vi "go2 -o.vi"() -> ()   [LabVIEW 2016]
uses:
  Classes/Controller/Motion/A3200 Folder/A3200.lvclass
  D:/Gantry_General/Classes/Controller/Motion/Motion Folder/Motion.lvclass
  Classes/Controller/Dispenser/Ultimus V2 Folder/Ultimus V2.lvclass
  Classes/Controller/I-O/NI-DAQ Folder/NI-DAQ.lvclass
  Classes/Controller/Motion/Motion Folder/Motion.lvclass
  Classes/Controller/I-O/I-O Folder/I-O.lvclass
  Classes/Controller/Dispenser/Dispenser Folder/Dispenser.lvclass
  <vilib>/Utility/file.llb/Read Delimited Spreadsheet (DBL).vi
panel:
  in  "controller in":T1
  out "draw point Cluster":T2
  in  "go patten":bool
  in  "tool go":bool
  in  "Tab Control":T3(tab)
  in  "XY go":bool
  in  "Z move to zero":bool
  in  "gule distances":dbl[](array[numeric])=[-0.6]
  out "needle XYZTheta In":dbl[](array[numeric])=[735.0, 1000.0, 55.0, 0.0]
  in  "needle xy":dbl[](array[numeric])=[735.0, 1000.0]
  in  "move to needle position":bool
  in  "XY":dbl[](array[numeric])=[1209.23, 800.59]
  in  "Camera to assembly center":bool
  in  "Camera sensor center":dbl[](array[numeric])=[1017.9301336735598, 802.7343660518175]
  in  "Camera to sensor center":bool
  in  "sensor angle":dbl=0.574830155359412
  in  "get sensor center":bool
  in  "get assembly center":bool
  in  "Syringe offset":dbl[](array[numeric])=[-219.555, -67.964]
  in  "Camera assembly center":dbl[](array[numeric])=[988.4421979205747, 1092.915302669506]
  in  "Syringe to assembly center":bool
  out "Syringe CAD center":dbl[](array[numeric])=[768.8871979205746, 1024.951302669506]
  in  "assembly angle":dbl=0.8050892331369087
  in  "get Syringe offset":bool
  in  "P0 on Delay":dbl=0.3 caption="Delay Time (s)"
  in  "new/data":bool
  in  "Vacuum Setting (0000)":i64 min=0 max=1000 step=1 format="%04.0f"
  in  "dispense change status":bool
  in  "Pressure":i16=30
  in  "on Delay":dbl=0.3 caption="Delay Time (s)"
  in  "off time":dbl=500.0
  in  "y":dbl=1.0
  out "delay off time":dbl=0.839
  in  "IO on /off":bool
  in  "Indices":i32[](array[numeric])=[11]
  in  "Values":bool[](array[boolean])=[FALSE]
  out "subarray":bool[](array[boolean])
  in  "baseplate thickness":dbl
  in  "Gule thickness":dbl
  in  "Sensor thickness":dbl
  in  "tool height":dbl
  in  "PCB thickness":dbl
  in  "file path (dialog if empty)":path=path "D:/Gantry_General/Main/ms_kao/data/CAD patten/CAD PCB full 0.8 P30 20210608/CAD PCB full 0.8 P30 20210608.txt"
  in  "Z height":dbl
  out "save data path":path=path "D:/Gantry_General/Main/ms_kao/data/CAD patten/CAD PCB full 0.8 P30 20210608/time/time20210712-164503.825.txt"
  out "folder and file name Cluster":T4={"Path"=path "D:/Gantry_General/Main/ms_kao/data/CAD patten/CAD PCB full 0.8 P30 20210608", "folder name"="time", "file name"="time", "extension"="txt", "add time string"=FALSE}
  out "i":i32=74
  out "size(s)":i32=75
  in  "stop":bool
  in  "go CAD":bool
  in  "new/data speed":bool
  in  "XY new Speed":dbl=25.0
  # "點膠速度"
  # "設定新速度"
  # "使用新/資料速度"
  # "間距70 mm"
  # "(1050, 865)\n(1050, 935)\n(1050,1005)"
  # "(910, 865)\n(910, 935)\n(910,1005)"
  # "(980, 865)\n(980, 935)\n(980,1005)"
  # "(840, 865)\n(840, 935)\n(840,1005)"
  # "9.5mm"
  # "0.32mm"
  # "0.2mm"
  # "0.1mm"
  # "0.1mm"
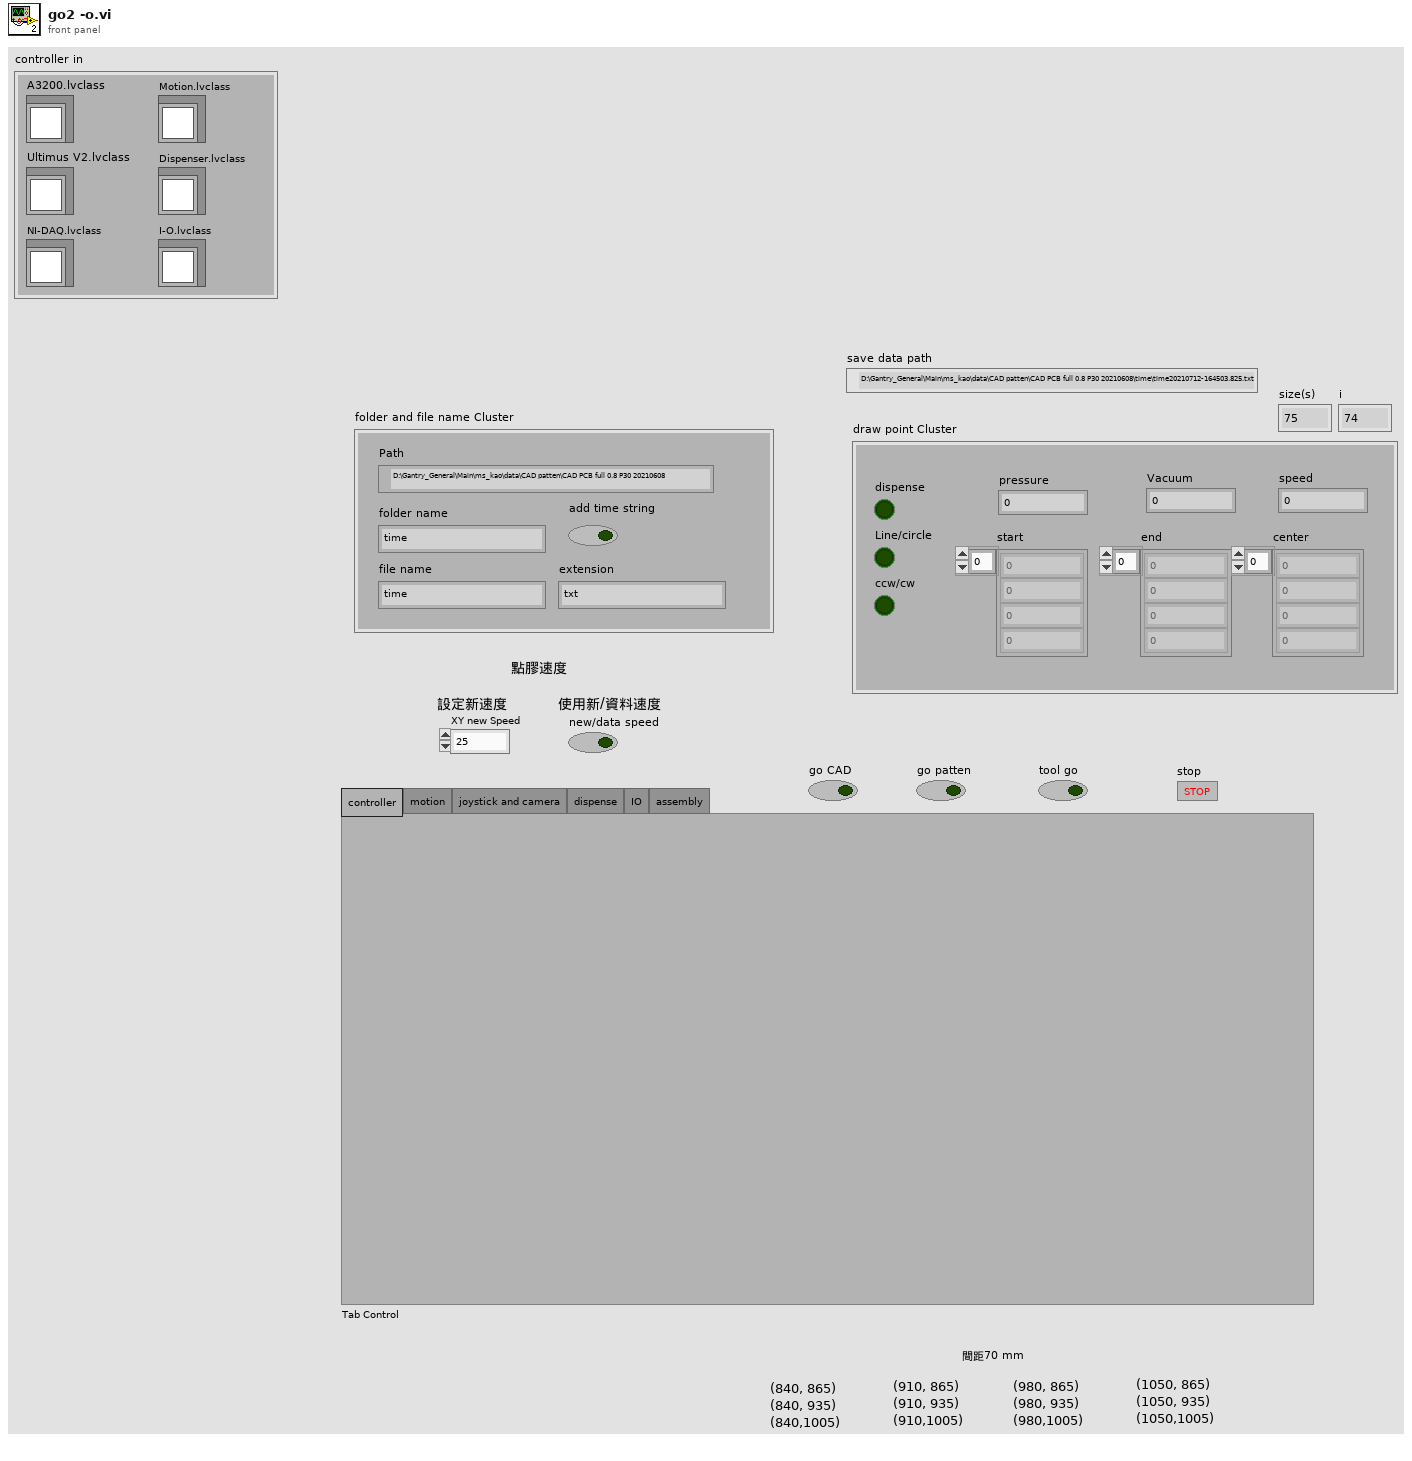
[diagram p1: front panel]
types:
  T1 = cluster{"A3200.lvclass":refnum<class "A3200.lvclass">, "Ultimus V2.lvclass":refnum<class "Ultimus V2.lvclass">, "NI-DAQ.lvclass":refnum<class "NI-DAQ.lvclass">, "Motion.lvclass":refnum<class "Motion.lvclass">, "I-O.lvclass":refnum<class "I-O.lvclass">, "Dispenser.lvclass":refnum<class "Dispenser.lvclass">}
  T2 = cluster{"dispense":bool, "Line/circle":bool, "ccw/cw":bool, "pressure":dbl, "speed":dbl, "start":dbl[], "end":dbl[], "center":dbl[], "Vacuum":dbl}
  T3 = enum32{"controller", "motion", "joystick and camera", "dispense", "IO", "assembly"}
  T4 = cluster{"Path":path, "folder name":string, "file name":string, "extension":string, "add time string":bool}
  T5 = cluster{"dispense":bool, "Line/circle":bool, "ccw/cw":bool, "pressure":dbl, "speed":dbl, "start":dbl[], "end":dbl[], "center":dbl[], "Vacuum":dbl}[]
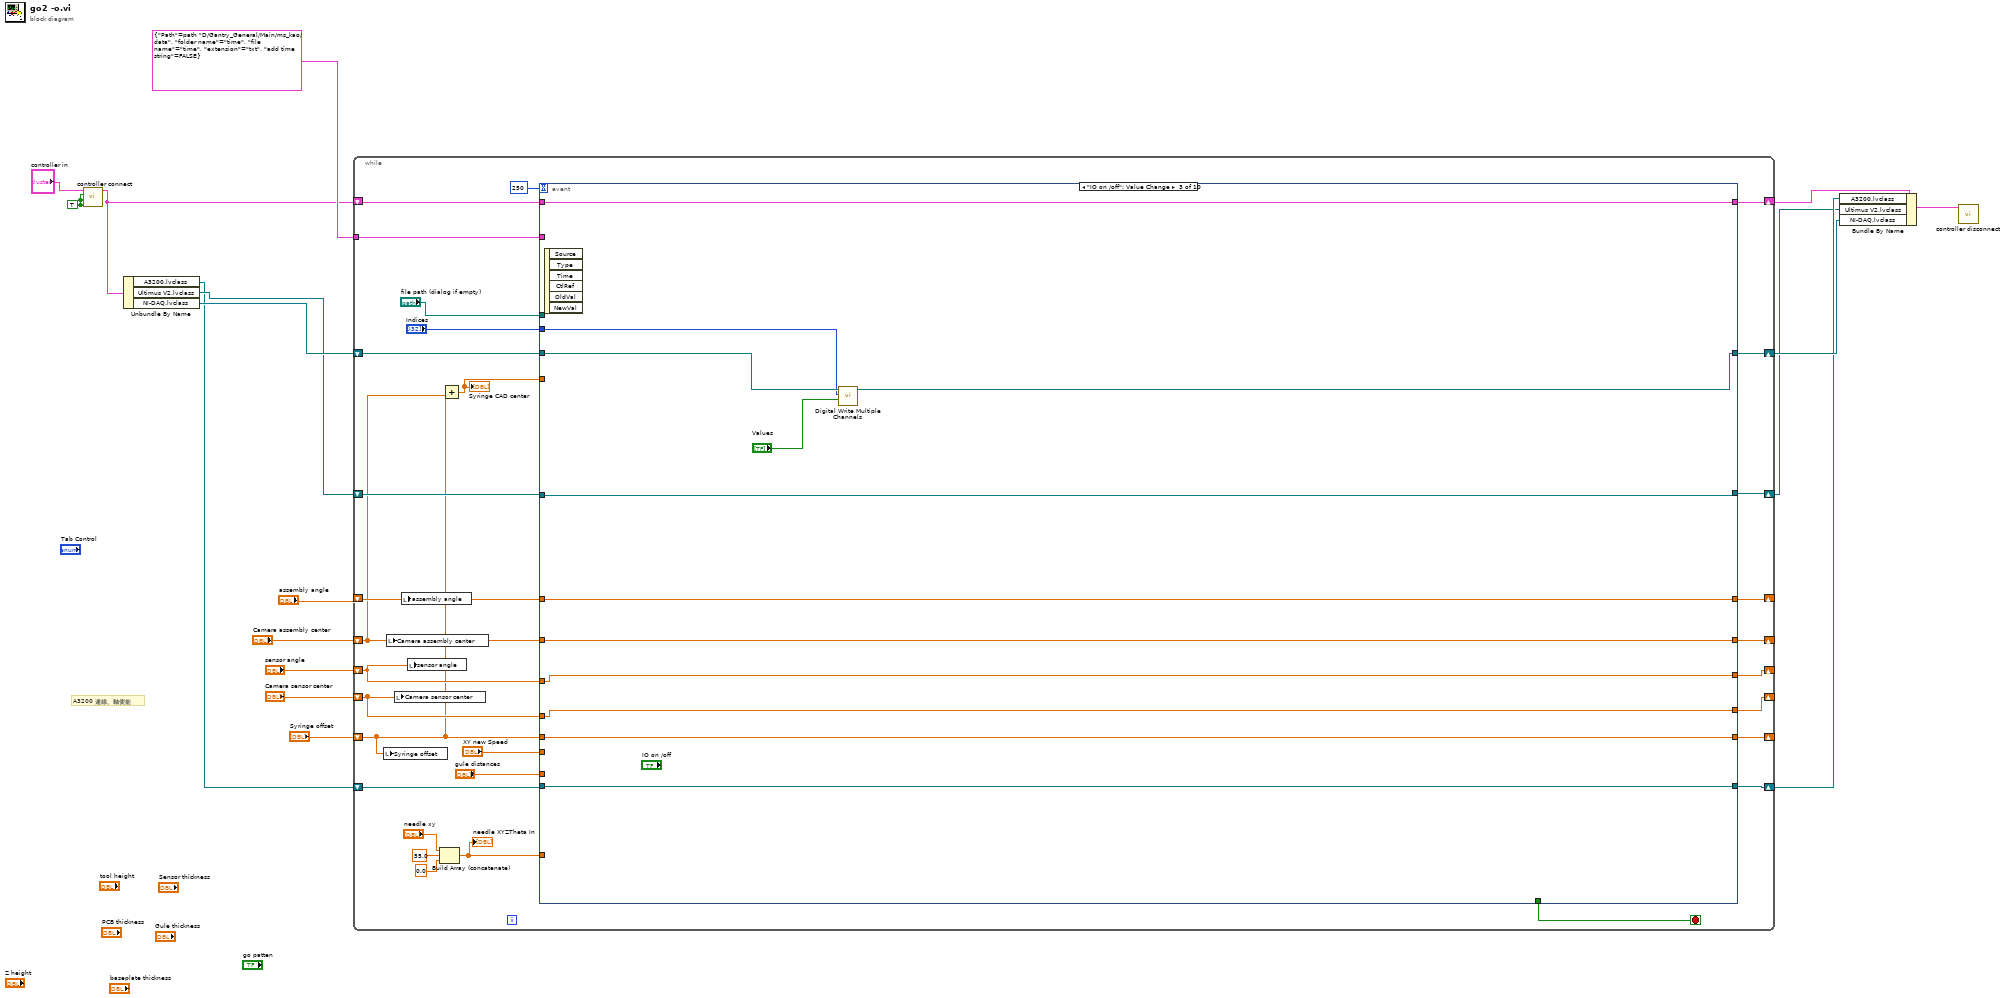
[diagram p0: block diagram]
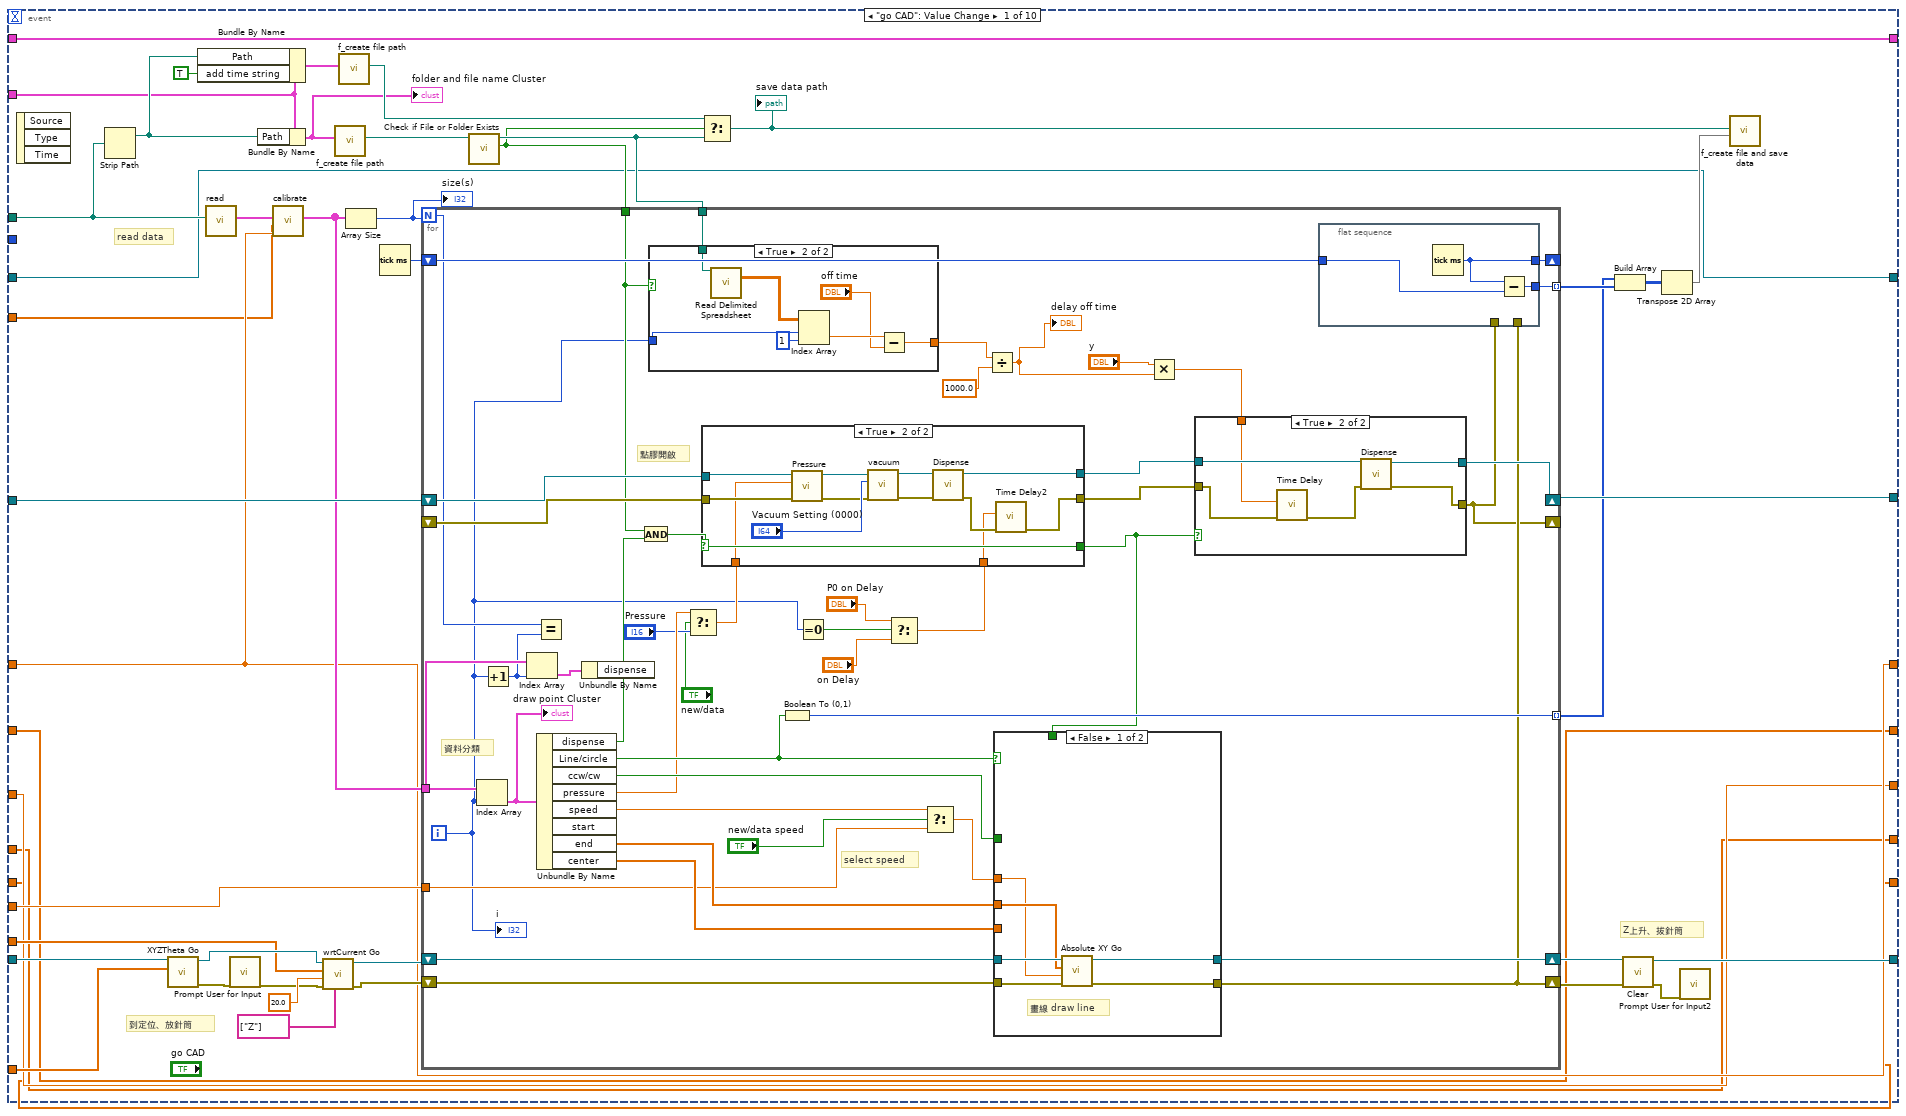
[diagram p2: hidden frame]
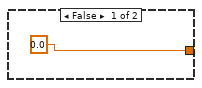
[diagram p3: hidden frame]
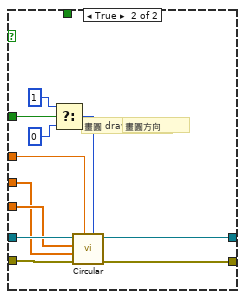
[diagram p6: hidden frame]
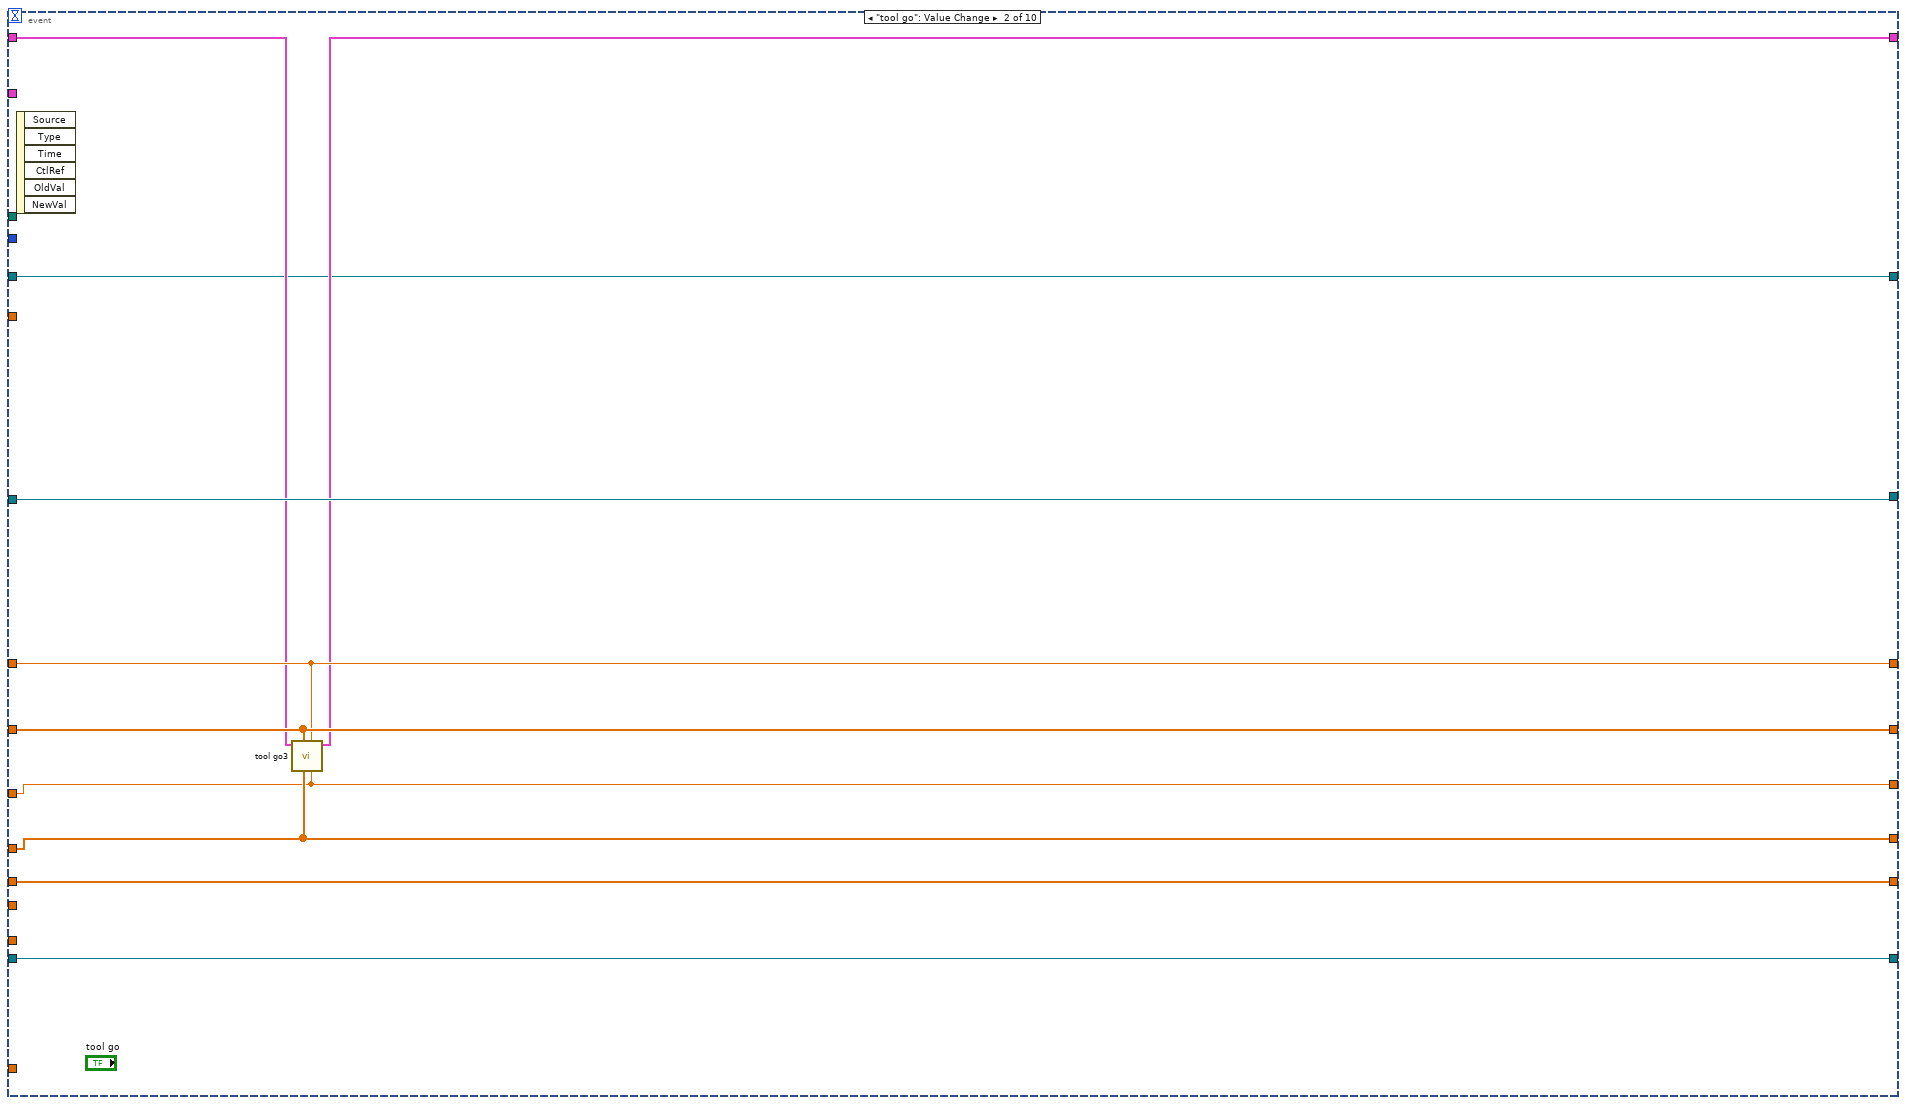
[diagram p7: hidden frame]
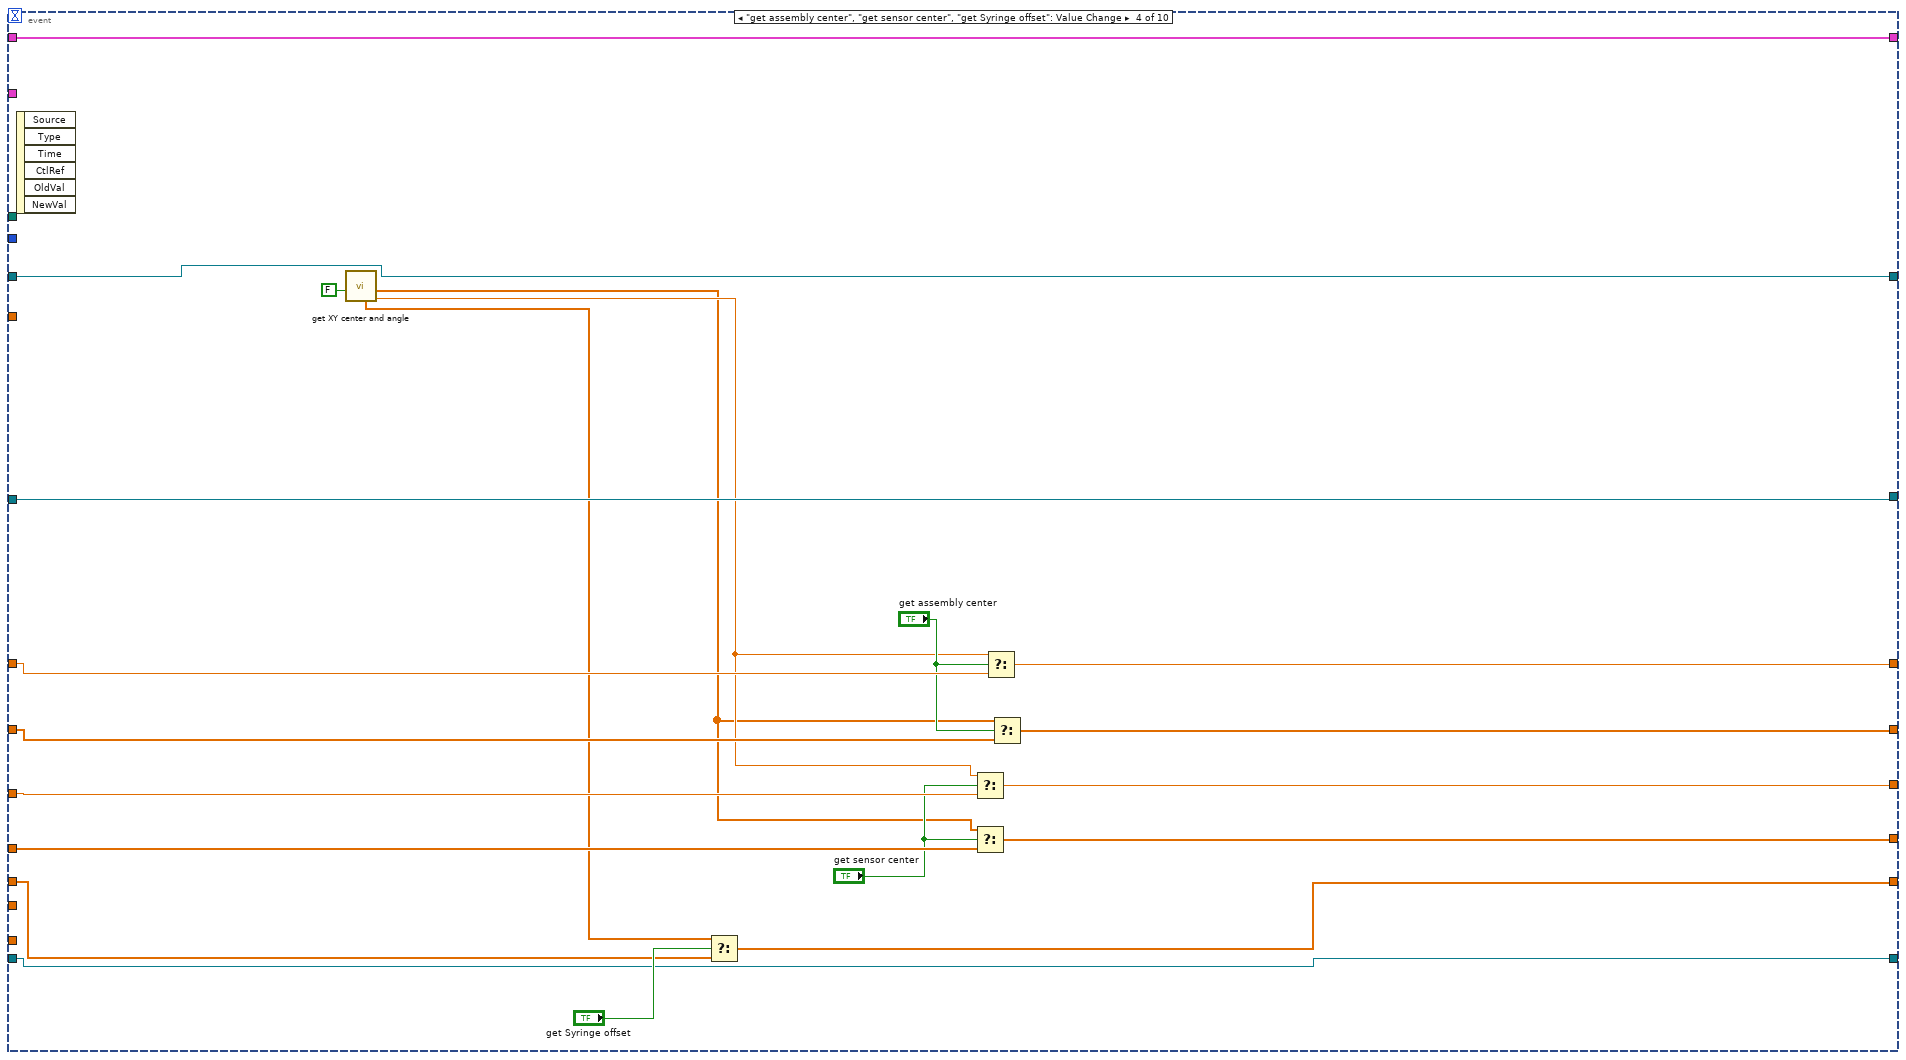
[diagram p8: hidden frame]
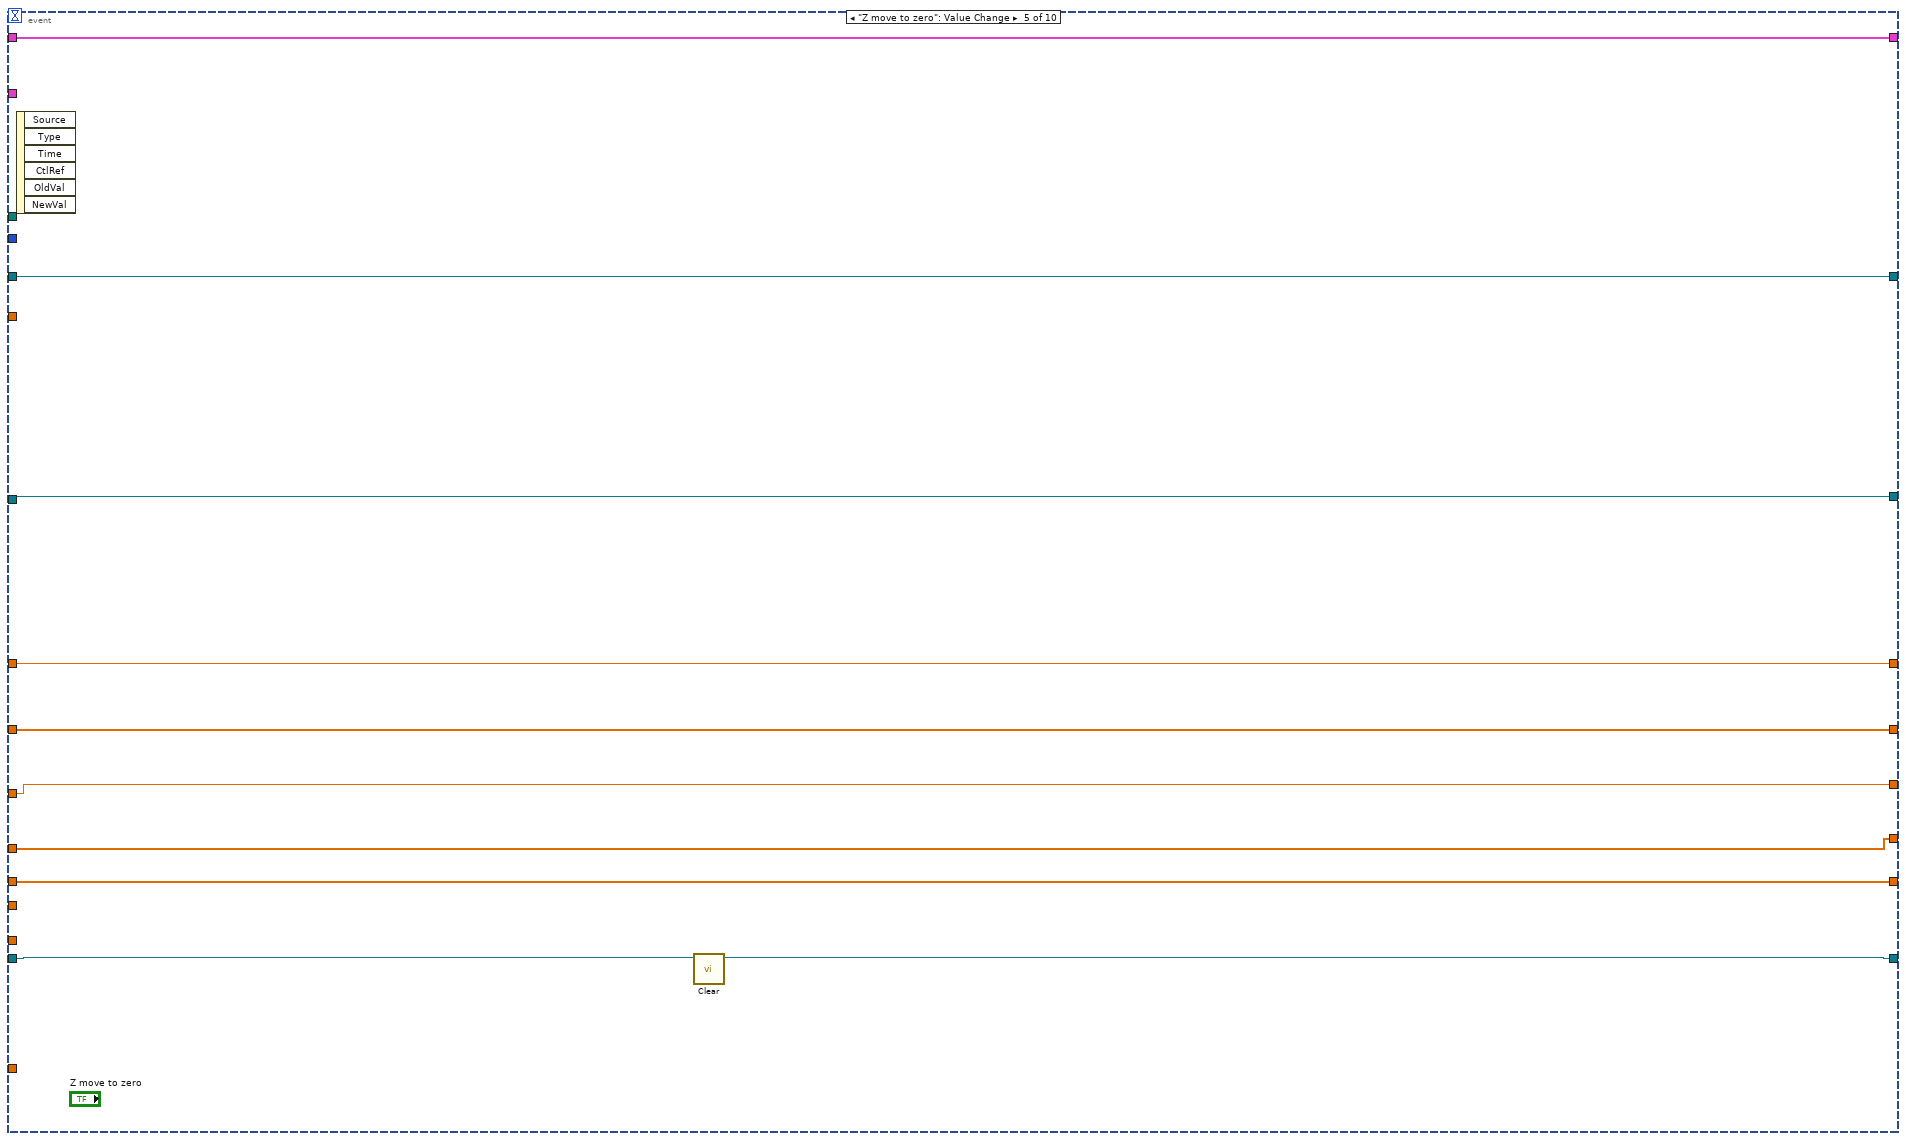
[diagram p9: hidden frame]
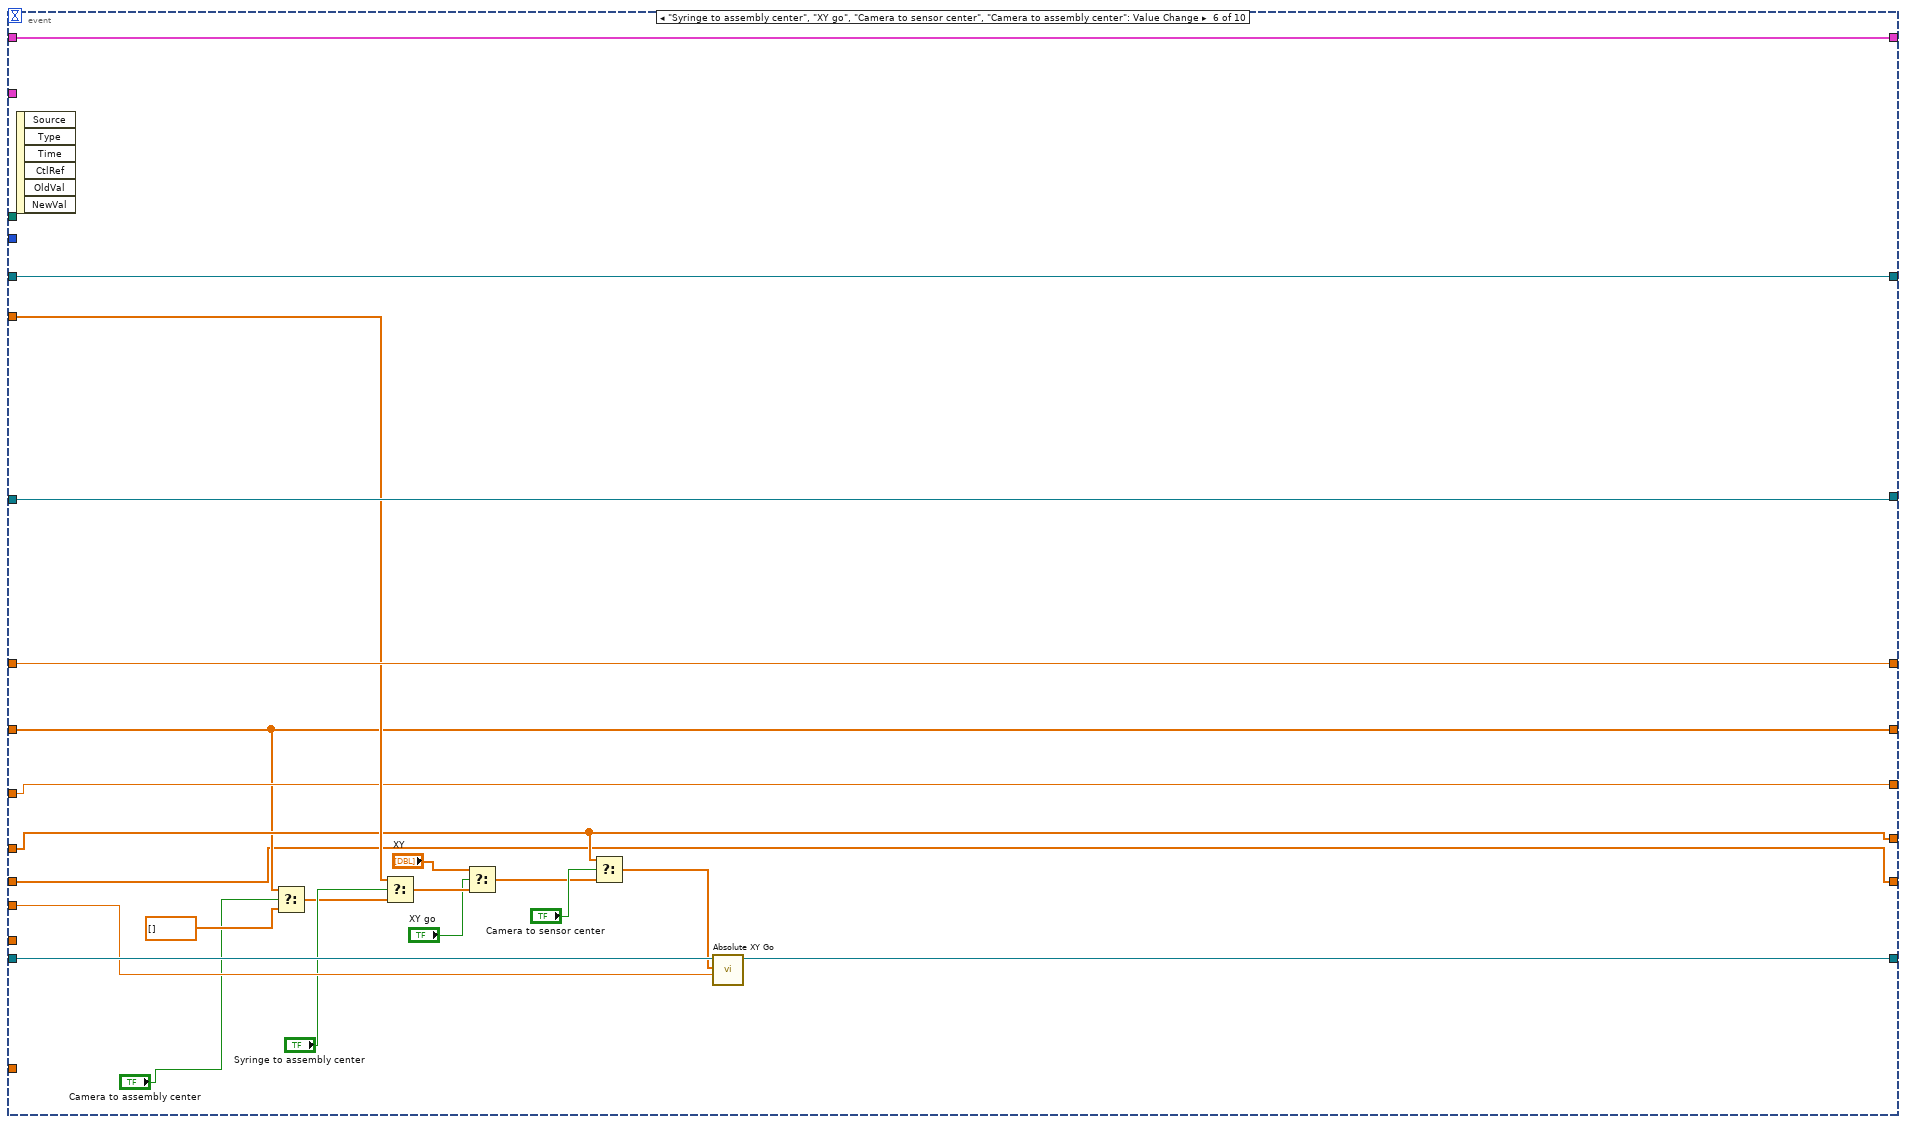
[diagram p10: hidden frame]
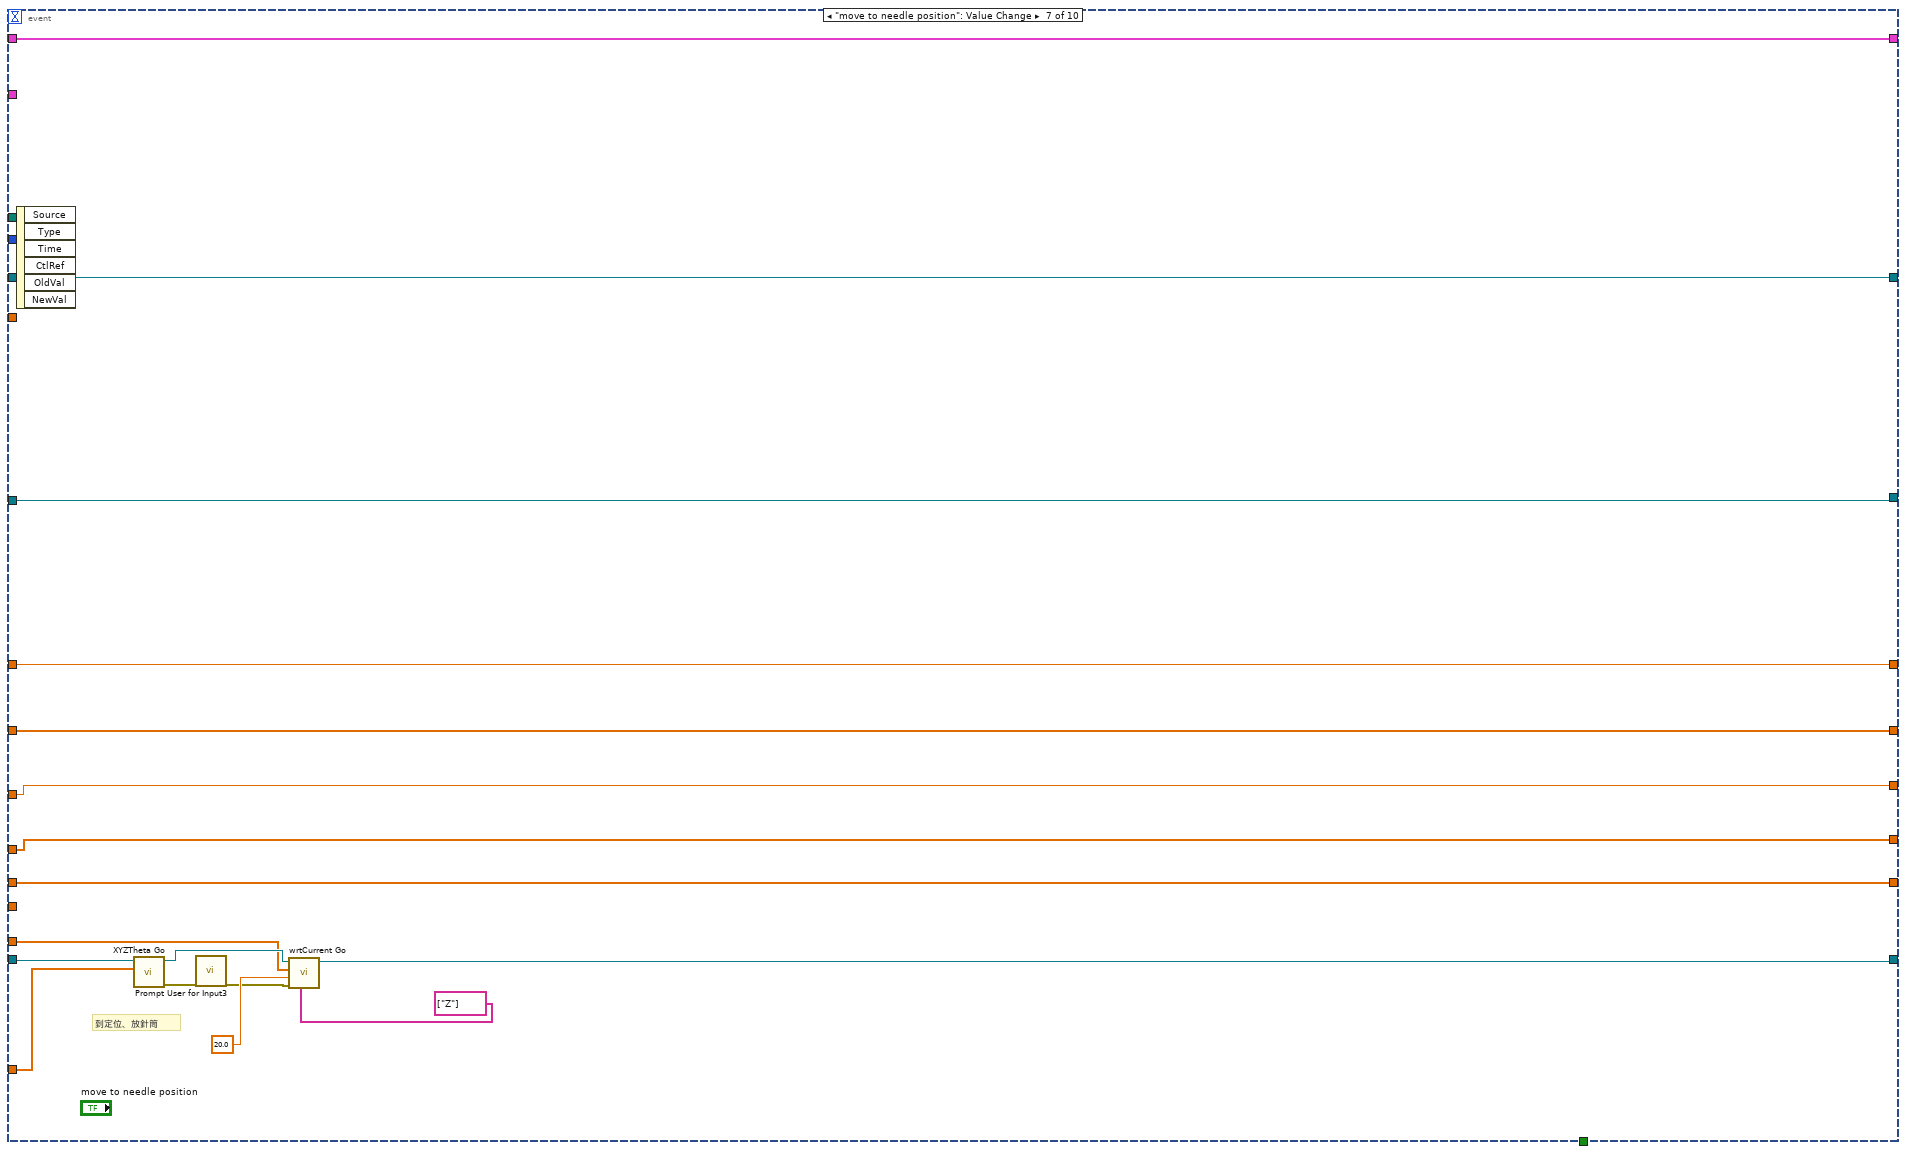
[diagram p11: hidden frame]
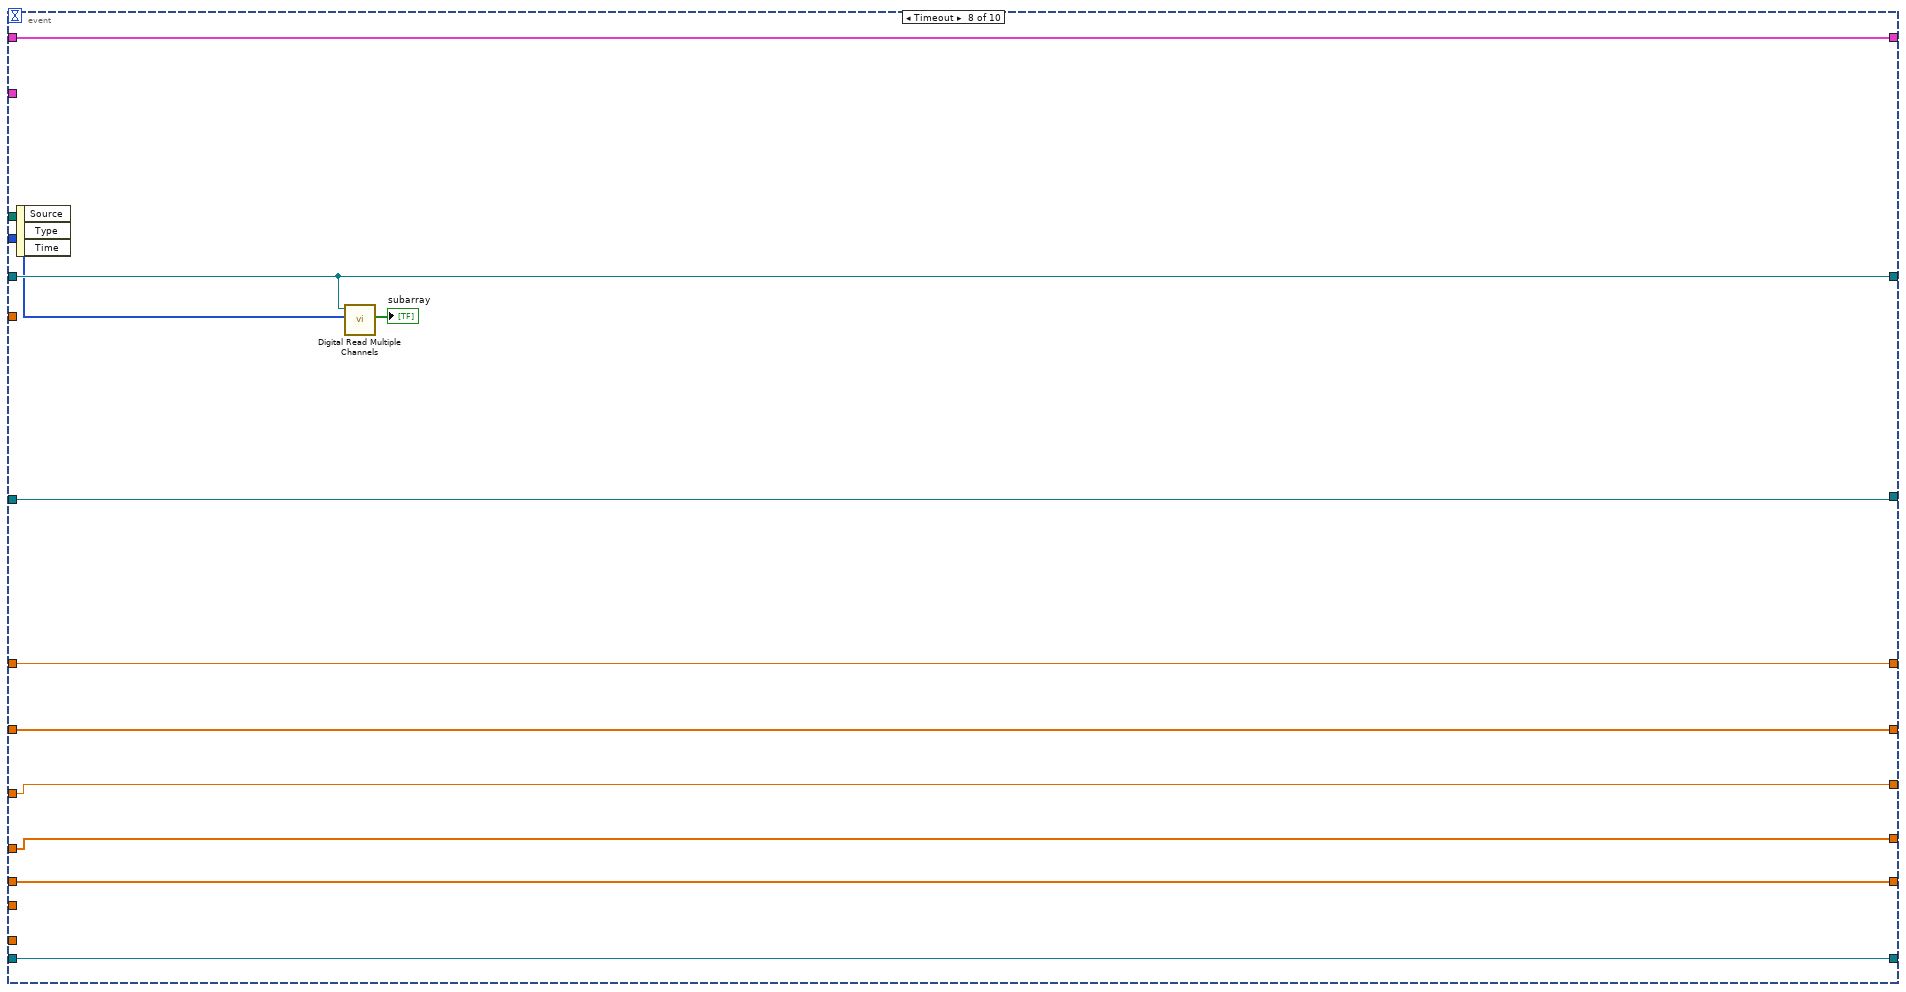
[diagram p12: hidden frame]
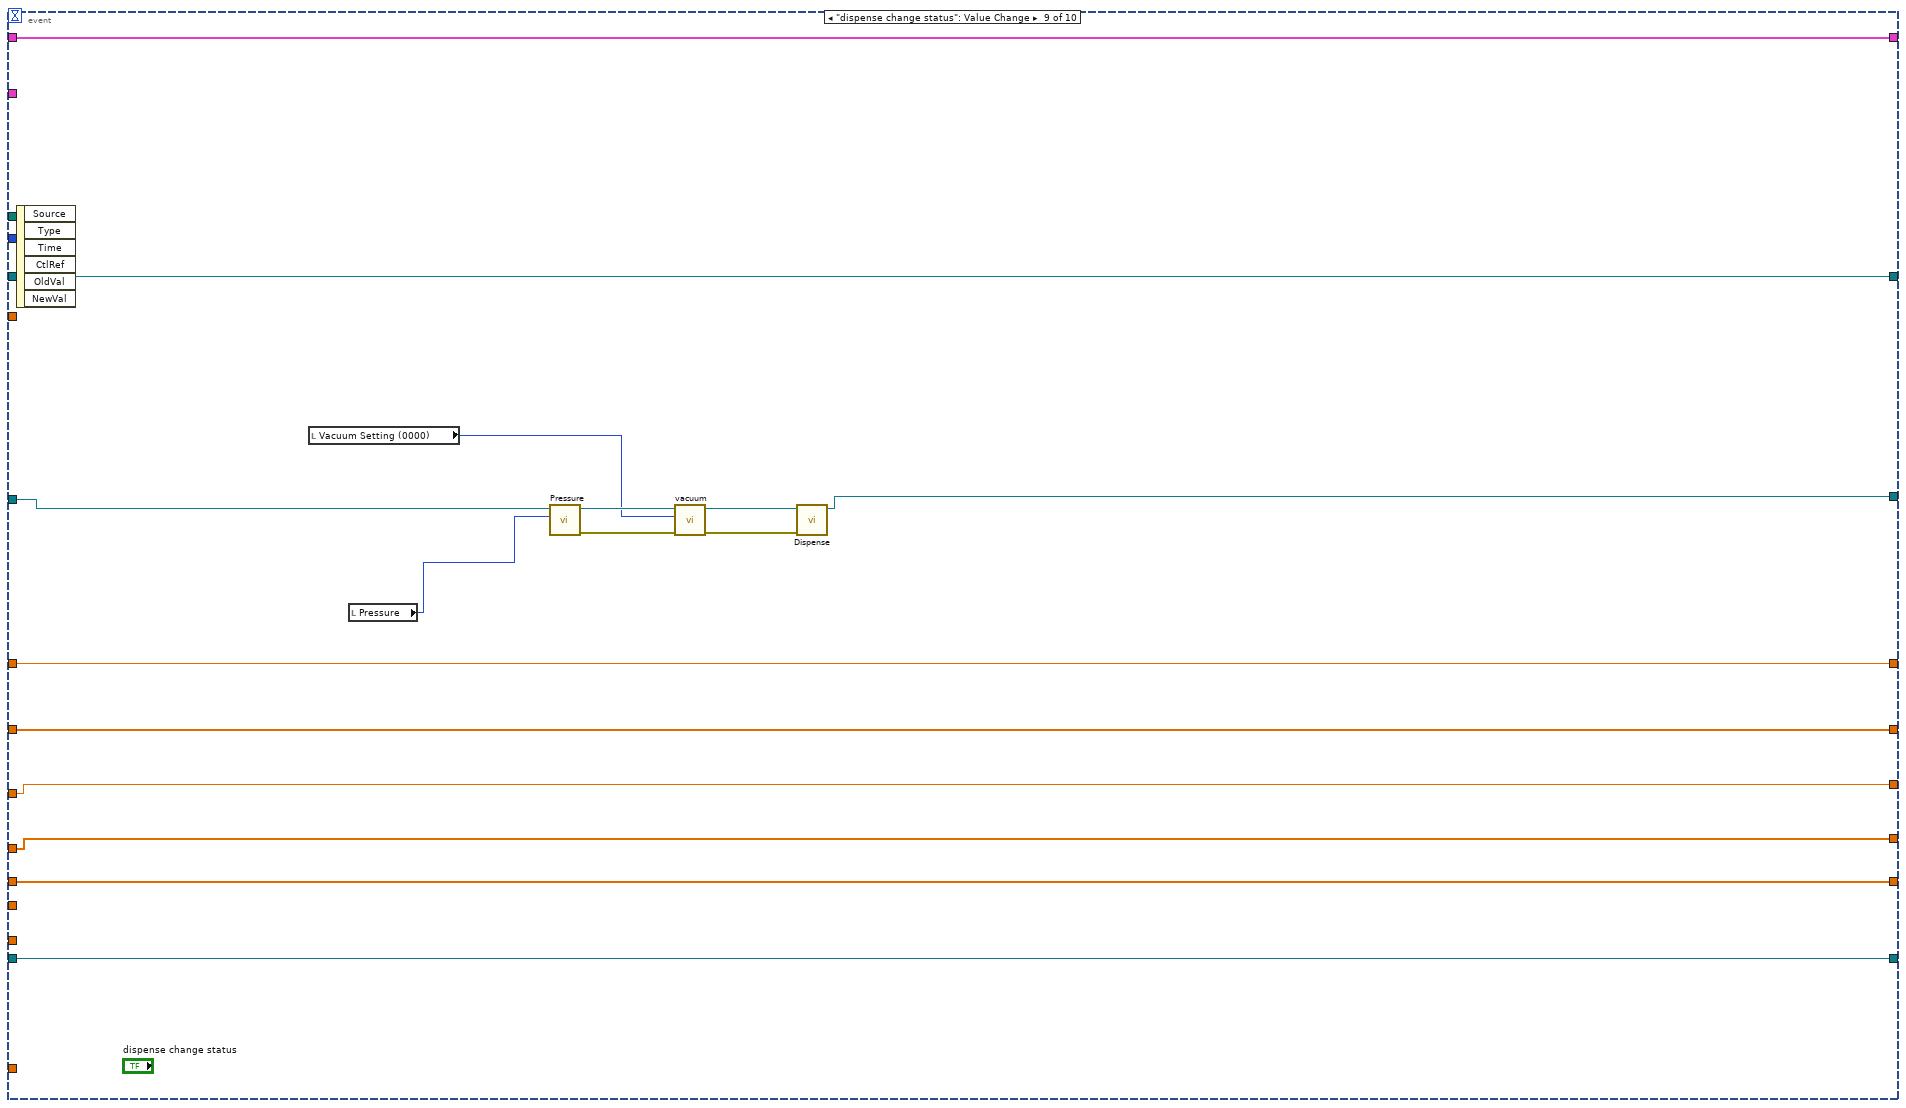
[diagram p13: hidden frame]
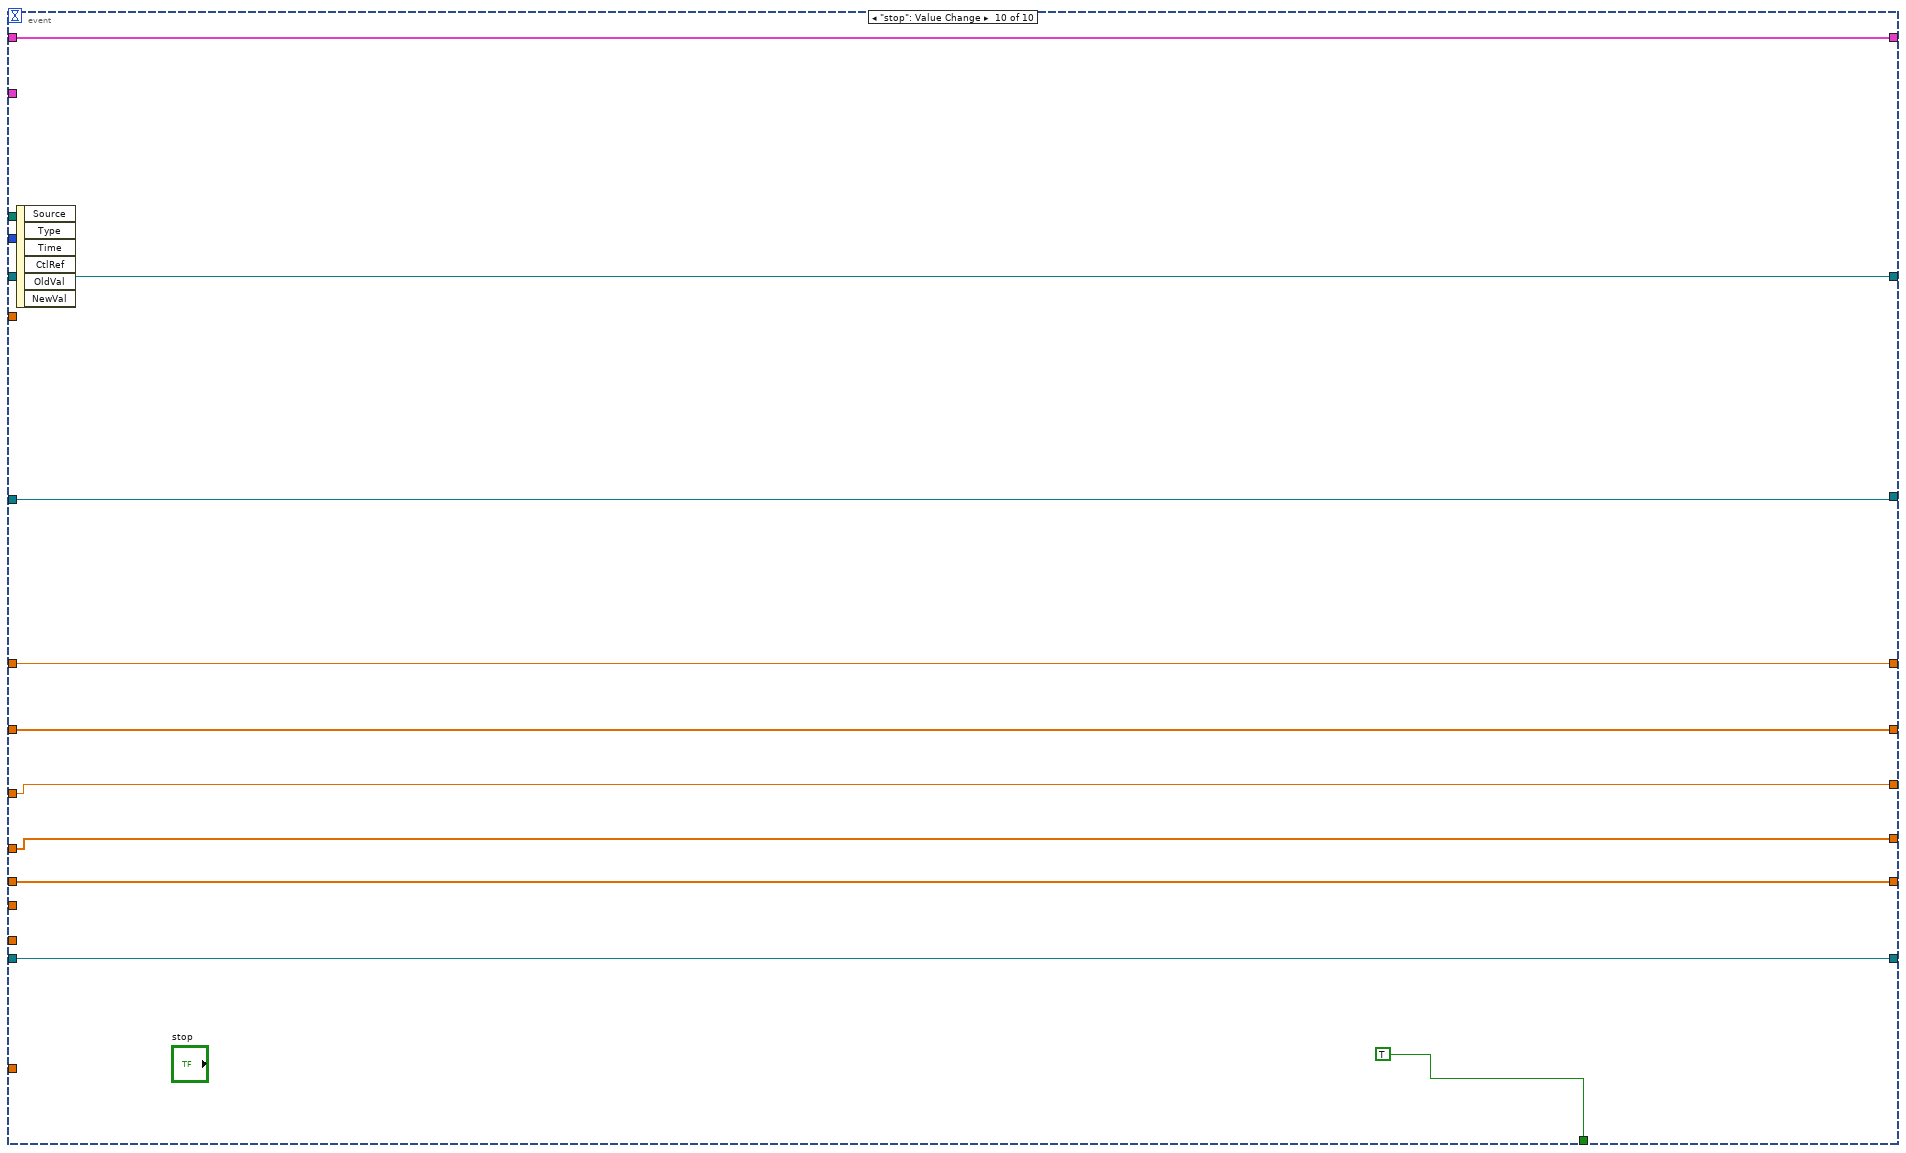
[diagram p14: hidden frame]
diagram:
  w10 = TRUE ("IO on")
  # "A3200 連線、軸使能"
  n1 = call "controller connect.vi"("IO on"=w10, "dispencer on"=w10, "motion on"=w10, "controller in"="controller in") -> ("controller out"=w6:T1)  [unwired: 7 in]
  n2 = Unbundle By Name(w6) -> ("A3200.lvclass"=w7:refnum<class "A3200.lvclass">, "Ultimus V2.lvclass"=w8:refnum<class "Ultimus V2.lvclass">, "NI-DAQ.lvclass"=w9:refnum<class "NI-DAQ.lvclass">)
  n3 = while {
    tunnel: T4 {"Path"=path "D:/Gantry_General/Main/ms_kao/data", "folder name"="time", "file name"="time", "extension"="txt", "add time string"=FALSE} ("folder and file name Cluster") -> [w39]
    shift-right: [w34] -> _
    shift-left: "assembly angle" -> [w29]
    shift-right: [w35] -> _
    shift-left: "Camera assembly center" -> [w28]
    shift-right: [w19] -> w3
    shift-left: w9 -> [w36]
    shift-right: [w30] -> _
    shift-left: "Camera sensor center" -> [w26]
    shift-right: [w31] -> _
    shift-left: "sensor angle" -> [w27]
    shift-right: [w25] -> _
    shift-left: "Syringe offset" -> [w24]
    shift-right: [w22] -> w2
    shift-left: w7 -> [w45]
    shift-right: [w18] -> w1
    shift-left: w8 -> [w46]
    shift-right: [w20] -> w4
    shift-left: w6 -> [w21]
    stop <- w47 stop-if-true
    n4 = local write "Syringe offset"(w24) -> ()
    n5 = local write "Camera assembly center"(w28) -> ()
    n6 = local write "Camera sensor center"(w26) -> ()
    n7 = local write "assembly angle"(w29) -> ()
    n8 = local write "sensor angle"(w27) -> ()
    n9 = Build Array (concatenate)("needle xy", 55.0, 0.0 ("element")) -> (w43:dbl[])
    "needle XYZTheta In" <- w43
    n10 = Add(x=w24, y=w28) -> (x+y=w33:dbl[])
    "Syringe CAD center" <- w33
    n11 = event shown="[2] \"IO on /off\": Value Change" {
      selector: _ -> [_ _ _ _ _ _ _ _ _ _]
      dyn-events: _ -> [_ _ _ _ _ _ _ _ _ _]
      timeout: 250 -> [_ _ _ _ _ _ _ _ _ _]
      tunnel: w45 -> [w87 w193 w209 w212 w242 w264 w277 w289 w301 w317]
      tunnel: [w78 w193 w209 w212 w241 w263 w273 w289 w301 w317] -> w22
      tunnel: w46 -> [w90 w199 w208 w232 w240 w261 w272 w292 w305 w316]
      tunnel: [w89 w199 w208 w232 w240 w261 w272 w292 w308 w316] -> w18
      tunnel: [_ _ _ _ _ _ _ _ _ TRUE] -> w47
      tunnel: w43 -> [w71 _ _ _ _ _ w276 _ _ _]
      tunnel: "gule distances" -> [w70 _ _ _ _ _ w275 _ _ _]
      tunnel: w29 -> [w56 w197 w210 w229 w239 w260 w271 w291 w300 w315]
      tunnel: w39 -> [w62 _ _ _ _ _ _ _ _ _]
      tunnel: "XY new Speed" -> [w57 _ _ _ _ w262 _ _ _ _]
      tunnel: w28 -> [w55 w198 w211 w228 w238 w247 w270 w290 w299 w314]
      tunnel: w36 -> [w48 w190 w207 w213 w233 w243 w265 w287 w293 w309]
      tunnel: [w55 w198 w211 w231 w238 w247 w270 w290 w299 w314] -> w35
      tunnel: [w56 w197 w210 w230 w239 w260 w271 w291 w300 w315] -> w34
      tunnel: w33 -> [w54 _ _ _ _ w258 _ _ _ _]
      tunnel: "Indices" -> [_ _ w205 _ _ _ _ w286 _ _]
      tunnel: [w53 w195 w204 w226 w237 w254 w269 w285 w298 w313] -> w31
      tunnel: [w52 w196 w203 w225 w236 w250 w268 w284 w297 w312] -> w30
      tunnel: w27 -> [w53 w195 w204 w224 w237 w254 w269 w285 w298 w313]
      tunnel: w26 -> [w52 w196 w203 w223 w236 w250 w268 w284 w297 w312]
      tunnel: w24 -> [w51 w194 w202 w217 w235 w245 w267 w283 w296 w311]
      tunnel: [w51 w194 w202 w216 w235 w245 w267 w283 w296 w311] -> w25
      tunnel: "file path (dialog if empty)" -> [w50 _ _ _ _ _ _ _ _ _]
      tunnel: w21 -> [w49 w192 w201 w214 w234 w244 w266 w282 w294 w310]
      tunnel: [w49 w191 w201 w214 w234 w244 w266 w282 w294 w310] -> w20
      tunnel: [w48 w190 w200 w213 w233 w243 w265 w287 w293 w309] -> w19
      event "go CAD": Value Change {
        # "Z上升、拔針筒"
        # "到定位、放針筒"
        # "read data"
        n12 = event-data() -> ()  [unwired: 1 in, 3 out]
        n13 = Strip Path(path=w50) -> (stripped path=w64:path)  [unwired: 1 out]
        n14 = call "XYZTheta Go.vi"("XYZTheta In"=w71, "Motion in"=w87) -> ("error out"=w86:errorcluster, "Motion out"=w83:refnum<class "A3200.lvclass">)  [unwired: 7 in, 1 out]
        n15 = Bundle By Name(cluster=w62, "Path"=w64, "add time string"=TRUE) -> (w60:T4)
        n16 = call "read.vi"("file path (dialog if empty)"=w50) -> ("Array"=w75:T5)  [unwired: 9 in]
        n17 = call "Prompt User for Input"("error in (no error)"=w86) -> ("error out"=w81:errorcluster)  [unwired: 17 in, 1 out]
        n18 = Bundle By Name(cluster=w62, "Path"=w64) -> (w58:T4)
        "folder and file name Cluster" <- w58
        n19 = call "calibrate.vi"("angle"=w56, "CAD center"=w54, "Array 3"=w75) -> ("Array 2"=w72:T5)  [unwired: 8 in]
        n20 = call-dynamic "wrtCurrent Go.vi"("axis names"=string[] ["Z"], "error in (no error)"=w81, "Speed"=20.0, "distances"=w70, "A3200 in"=w83) -> ("error out"=w80:errorcluster, "A3200 out"=w82:refnum<class "A3200.lvclass">)  [unwired: 5 in]
        n21 = call "f_create file path.vi"("folder and file name Cluster"=w58) -> ("appended path"=w67:path)  [unwired: 10 in]
        n22 = call "f_create file path.vi"("folder and file name Cluster"=w60) -> ("appended path"=w61:path)  [unwired: 10 in]
        n23 = Array Size(array=w72) -> (size(s)=w73:i32)
        "size(s)" <- w73
        n24 = Tick Count (ms)() -> (millisecond timer value=w68:u32)
        n25 = call <vilib>:"Check if File or Folder Exists.vi"("path"=w67) -> ("file or folder exists?"=w59:bool, "dup path"=w65:path)  [unwired: 8 in, 1 out]
        n26 = for {
          N: w73 -> [w105]
          shift-right: [w111] -> w77
          shift-left: w80 -> [w137]
          shift-right: [w135] -> w79
          shift-left: w82 -> [w136]
          shift-right: [w127] -> _
          shift-left: w68 -> [w128]
          tunnel: [w126] -> w91 mode=indexing
          shift-right: [w124] -> w89
          shift-left: w90 -> [w120]
          shift-right: [w110] -> _
          shift-left: _ -> [w119]
          tunnel: [w121] -> w74 mode=indexing
          tunnel: w72 -> [w107]
          tunnel: w59 -> [w115]
          tunnel: w65 -> [w116]
          tunnel: w57 -> [w103]
          i -> [w93]
          # "點膠開啟"
          # "select speed"
          # "資料分類"
          n27 = Index Array(array=w107, index=w93) -> (element=w92:T2)
          "draw point Cluster" <- w92
          n28 = Increment(x=w93) -> (x+1=w106:i32)
          n29 = Index Array(array=w107, index=w106) -> (element=w108:T2)
          n30 = Equal?(x=w105, y=w106) -> ()  [unwired: 1 out]
          n31 = Unbundle By Name(w92) -> ("dispense"=w117:bool, "Line/circle"=w122:bool, "ccw/cw"=w132:bool, "pressure"=w100:dbl, "speed"=w131:dbl, "end"=w134:dbl[], "center"=w133:dbl[])  [unwired: 1 out]
          n32 = Unbundle By Name(w108) -> ()  [unwired: 1 out]
          n33 = And(x=w115, y=w117) -> (x .and. y?=w118:bool)
          n34 = case shown="True" w115 {
            tunnel: w116 -> [_ w147]
            tunnel: w93 -> [_ w146]
            tunnel: [0.0 ("Numeric") w142] -> w102
            frame False {
            }
            frame True {
              n35 = call-poly <vilib>:"Read Delimited Spreadsheet.vi"("file path (dialog if empty)"=w147) -> ("all rows"=w148:dbl[][])  [unwired: 9 in, 5 out]
              n36 = Index Array(array=w148, index (row)=w146, index (col)=1 ("disabled index (col)")) -> (element=w144:dbl)
              n37 = Subtract(x=w144, y="off time") -> (x-y=w142:dbl)
            }
          }
          n38 = Select(t=w100, s="new/data", f="Pressure") -> (s? t:f=w101:dbl)
          n39 = Boolean To (0,1)(Boolean=w122) -> (0, 1=w121:i16)
          n40 = Equal To 0?(x=w93) -> (x = 0?=w94:bool)
          n41 = Select(t="P0 on Delay", s=w94, f="on Delay") -> (s? t:f=w95:dbl)
          n42 = case shown="True" w118 {
            selector: w118 -> [w159 w171]
            tunnel: [w158 w172] -> w125
            tunnel: [w159 w171] -> w104
            tunnel: w120 -> [w158 w166]
            tunnel: w119 -> [w157 w165]
            tunnel: [w157 w169] -> w123
            tunnel: w101 -> [_ w161]
            tunnel: w95 -> [_ w160]
            frame False {
            }
            frame True {
              n43 = call-dynamic "Pressure.vi"("error in (no error)"=w165, "Pressure"=w161, "Ultimus V in"=w166) -> ("error out"=w164:errorcluster, "Ultimus V out"=w167:refnum<class "Ultimus V2.lvclass">)  [unwired: 7 in]
              n44 = call "vacuum.vi"("error in (no error)"=w164, "Vacuum Setting (0000)"="Vacuum Setting (0000)", "Ultimus V in"=w167) -> ("error out"=w163:errorcluster, "Ultimus V out"=w162:refnum<class "Ultimus V2.lvclass">)  [unwired: 7 in]
              n45 = call-dynamic "Dispense.vi"("error in (no error)"=w163, "Ultimus V in"=w162) -> ("error out"=w170:errorcluster, "Ultimus V out"=w172:refnum<class "Ultimus V2.lvclass">)  [unwired: 8 in]
              n46 = call "Time Delay2"("error in (no error)"=w170, "Delay Time (s)"=w160) -> ("error out"=w169:errorcluster)  [unwired: 9 in]
            }
          }
          n47 = Select(t=w131, s="new/data speed", f=w103) -> (s? t:f=w130:dbl)
          n48 = Divide(x=w102, y=1000.0) -> (x/y=w113:dbl)
          "delay off time" <- w113
          n49 = case shown="False" w122 {
            tunnel: [w177 w189] -> w111
            tunnel: w137 -> [w178 w188]
            tunnel: w136 -> [w176 w187]
            tunnel: [w175 w186] -> w135
            tunnel: w134 -> [w174 w184]
            tunnel: w133 -> [_ w185]
            tunnel: w132 -> [_ w183]
            tunnel: w130 -> [w173 w179]
            tunnel: w104 -> [_ _]
            frame False {
              # "畫線 draw line"
              n50 = call-dynamic "Absolute XY Go.vi"("error in (no error)"=w178, "Speed"=w173, "XY"=w174, "Gantry in"=w176) -> ("error out"=w177:errorcluster, "Gantry out"=w175:refnum<class "A3200.lvclass">)  [unwired: 6 in]
            }
            frame True {
              # "畫圓方向"
              # "畫圓 draw circle"
              n51 = Select(t=1, s=w183, f=0) -> (s? t:f=w182:i32)
              n52 = call-dynamic "Circular.vi"("Direction"=w182, "Speed"=w179, "error in (no error)"=w188, "XY End"=w184, "XY Center"=w185, "Gantry in"=w187) -> ("error out"=w189:errorcluster, "Gantry out"=w186:refnum<class "A3200.lvclass">)  [unwired: 4 in]
            }
          }
          n53 = Multiply(x="y", y=w113) -> (x*y=w109:dbl)
          n54 = case shown="True" w104 {
            tunnel: [w150 w156] -> w124
            tunnel: w125 -> [w150 w155]
            tunnel: w123 -> [w149 w152]
            tunnel: [w149 w154] -> w110
            tunnel: w109 -> [_ w151]
            frame False {
            }
            frame True {
              n55 = call "Time Delay"("error in (no error)"=w152, "Delay Time (s)"=w151) -> ("error out"=w153:errorcluster)  [unwired: 9 in]
              n56 = call-dynamic "Dispense.vi"("error in (no error)"=w153, "Ultimus V in"=w155) -> ("error out"=w154:errorcluster, "Ultimus V out"=w156:refnum<class "Ultimus V2.lvclass">)  [unwired: 8 in]
            }
          }
          n57 = flat-sequence {
            tunnel: w128 -> [w140]
            tunnel: [w139] -> w127
            tunnel: [w138] -> w126
            tunnel: w111 -> [_]
            tunnel: w110 -> [_]
            frame #0 {
              n58 = Tick Count (ms)() -> (millisecond timer value=w139:u32)
              n59 = Subtract(x=w139, y=w140) -> (x-y=w138:u32)
            }
          }
          "i" <- w93
        }
        n60 = Select(t=w61, s=w59, f=w65) -> (s? t:f=w66:path)
        "save data path" <- w66
        n61 = Build Array(w74, w91) -> (w88:u32[][])
        n62 = call "Clear.vi"("error in (no error)"=w77, "Motion in"=w79) -> ("error out"=w76:errorcluster, "Motion out"=w78:refnum<class "A3200.lvclass">)  [unwired: 8 in]
        n63 = Transpose 2D Array(2D array=w88) -> (transposed array=w69:u32[][])
        n64 = call "Prompt User for Input2"("error in (no error)"=w76) -> ()  [unwired: 17 in, 2 out]
        n65 = call "f_create file and save data.vi"("2D data"=w69, "path"=w66) -> ()  [unwired: 9 in, 1 out]
      }
      event "tool go": Value Change {
        n66 = event-data() -> ()  [unwired: 1 in, 6 out]
        n67 = call "tool go3.vi"("sensor angle"=w195, "assembly angle"=w197, "sensor center"=w196, "assembly center"=w198, "controller in"=w192) -> ("controller out"=w191:T1)  [unwired: 5 in, 1 out]
      }
      event "IO on /off": Value Change {
        n68 = event-data() -> ()  [unwired: 1 in, 6 out]
        n69 = call-dynamic "Digital Write Multiple Channels.vi"("Values"="Values", "Indices"=w205, "NI-DAQ in"=w207) -> ("NI-DAQ out"=w200:refnum<class "NI-DAQ.lvclass">)  [unwired: 7 in, 1 out]
      }
      event "get assembly center", "get sensor center", "get Syringe offset": Value Change {
        n70 = event-data() -> ()  [unwired: 1 in, 6 out]
        n71 = call "get XY center and angle.vi"("output P1 XY"=FALSE) -> ("XY theta out"=w221:dbl, "XY center out"=w220:dbl[], "offset P1-P2"=w218:dbl[])  [unwired: 7 in, 1 out]
        n72 = Select(t=w218, s="get Syringe offset", f=w217) -> (s? t:f=w216:dbl[])
        n73 = Select(t=w221, s="get sensor center", f=w224) -> (s? t:f=w226:dbl)
        n74 = Select(t=w220, s="get sensor center", f=w223) -> (s? t:f=w225:dbl[])
        n75 = Select(t=w221, s="get assembly center", f=w229) -> (s? t:f=w230:dbl)
        n76 = Select(t=w220, s="get assembly center", f=w228) -> (s? t:f=w231:dbl[])
      }
      event "Z move to zero": Value Change {
        n77 = event-data() -> ()  [unwired: 1 in, 6 out]
        n78 = call "Clear.vi"("Motion in"=w242) -> ("Motion out"=w241:refnum<class "A3200.lvclass">)  [unwired: 9 in, 1 out]
      }
      event "Syringe to assembly center", "XY go", "Camera to sensor center", "Camera to assembly center": Value Change {
        n79 = event-data() -> ()  [unwired: 1 in, 6 out]
        n80 = Select(t=w247, s="Camera to assembly center", f=dbl[] []) -> (s? t:f=w248:dbl[])
        n81 = Select(t=w258, s="Syringe to assembly center", f=w248) -> (s? t:f=w257:dbl[])
        n82 = Select(t="XY", s="XY go", f=w257) -> (s? t:f=w252:dbl[])
        n83 = Select(t=w250, s="Camera to sensor center", f=w252) -> (s? t:f=w251:dbl[])
        n84 = call-dynamic "Absolute XY Go.vi"("Speed"=w262, "XY"=w251, "Gantry in"=w264) -> ("Gantry out"=w263:refnum<class "A3200.lvclass">)  [unwired: 7 in, 1 out]
      }
      event "move to needle position": Value Change {
        # "到定位、放針筒"
        n85 = event-data() -> ()  [unwired: 1 in, 6 out]
        n86 = call "XYZTheta Go.vi"("XYZTheta In"=w276, "Motion in"=w277) -> ("error out"=w281:errorcluster, "Motion out"=w279:refnum<class "A3200.lvclass">)  [unwired: 7 in, 1 out]
        n87 = call "Prompt User for Input3"("error in (no error)"=w281) -> ("error out"=w278:errorcluster)  [unwired: 17 in, 1 out]
        n88 = call-dynamic "wrtCurrent Go.vi"("axis names"=string[] ["Z"], "error in (no error)"=w278, "Speed"=20.0, "distances"=w275, "A3200 in"=w279) -> ("A3200 out"=w273:refnum<class "A3200.lvclass">)  [unwired: 5 in, 1 out]
      }
      event Timeout {
        n89 = event-data() -> ()  [unwired: 1 in, 3 out]
        n90 = call-dynamic "Digital Read Multiple Channels.vi"("Array"=w286, "NI-DAQ in"=w287) -> ("subarray"=→"subarray":bool[])  [unwired: 7 in, 2 out]
      }
      event "dispense change status": Value Change {
        n91 = event-data() -> ()  [unwired: 1 in, 6 out]
        n92 = local read "Vacuum Setting (0000)"() -> (w304:i64)
        n93 = local read "Pressure"() -> (w295:i16)
        n94 = call-dynamic "Pressure.vi"("Pressure"=w295, "Ultimus V in"=w305) -> ("error out"=w303:errorcluster, "Ultimus V out"=w306:refnum<class "Ultimus V2.lvclass">)  [unwired: 8 in]
        n95 = call "vacuum.vi"("error in (no error)"=w303, "Vacuum Setting (0000)"=w304, "Ultimus V in"=w306) -> ("error out"=w302:errorcluster, "Ultimus V out"=w307:refnum<class "Ultimus V2.lvclass">)  [unwired: 7 in]
        n96 = call-dynamic "Dispense.vi"("error in (no error)"=w302, "Ultimus V in"=w307) -> ("Ultimus V out"=w308:refnum<class "Ultimus V2.lvclass">)  [unwired: 8 in, 1 out]
      }
      event "stop": Value Change {
        n97 = event-data() -> ()  [unwired: 1 in, 6 out]
      }
    }
  }
  n98 = Bundle By Name(cluster=w4, "A3200.lvclass"=w2, "Ultimus V2.lvclass"=w1, "NI-DAQ.lvclass"=w3) -> (w5:T1)
  n99 = call "controller disconnect.vi"("controller 2"=w5) -> ()  [unwired: 11 in]
